vi "MyRIO Lidar Init.vi"(8 "error in (no error)":errorcluster) -> (0 "error out":errorcluster)   [LabVIEW 2017]
panel:
  out "Lidar index":i32
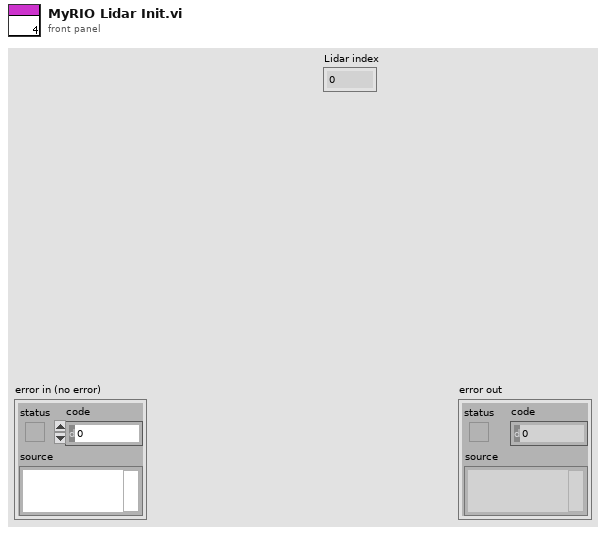
[diagram p1: front panel]
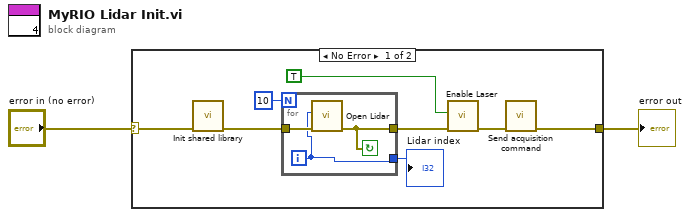
[diagram p0: block diagram]
diagram:
  n1 = case shown="No Error" "error in (no error)" {
    selector: "error in (no error)" -> [w10 w14]
    tunnel: [w5 w14] -> w1
    frame No Error {
      n2 = call "Init shared library.vi"("error in (no error)"=w10) -> ("error out"=w9:errorcluster)  [unwired: 10 in]
      n3 = for {
        N: 10 -> [_]
        tunnel: w9 -> [w13]
        tunnel: [w12] -> w8
        tunnel: [w11] -> w3
        i -> [w11]
        stop <- w12 continue-if-true
        n4 = call "Open Lidar.vi"("error in (no error)"=w13, "Lidar Number"=w11) -> ("error out"=w12:errorcluster)  [unwired: 9 in]
      }
      "Lidar index" <- w3
      n5 = call "Enable Laser.vi"("error in (no error)"=w8, "Enable Laser"=TRUE) -> ("error out"=w6:errorcluster)  [unwired: 9 in]
      n6 = call "Send acquisition command.vi"("error in (no error)"=w6) -> ("error out"=w5:errorcluster)  [unwired: 10 in]
    }
    frame Error {
    }
  }
  "error out" <- w1
